vi "Reset Generator.vi"(8 "error in (no error)":errorcluster, 10 "Waveform Generation (0:1)":u16(ring) items=["1", "2"], 11 "VISA resource name":refnum<visa-resource-name>) -> (0 "error out":errorcluster, 3 "VISA resource name out":refnum<visa-resource-name>)   [LabVIEW 2015, in "Agilent 2000 3000 X-Series.lvlib"]
doc: "Restores the waveform generator factory default settings (1 kHz sine wave, 500 mVpp, 0 V offset)."
uses:
  Agilent 2000 3000 X-Series.lvlib
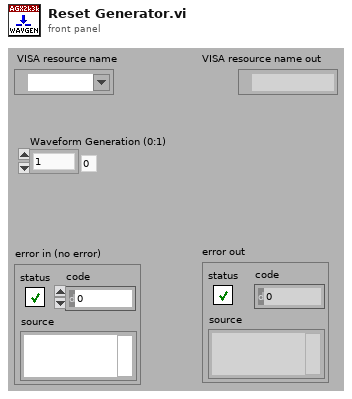
[diagram p1: front panel]
types:
  T1 = typedef "Agilent 2000 3000 X-Series.lvlib/Extended User Data.ctl" = cluster{"X-Series Mode":u16, "Acquisition Type (0: Normal)":i32}
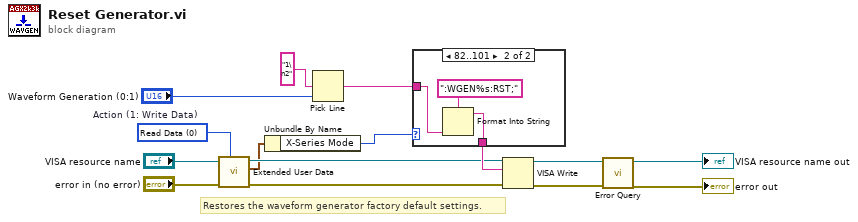
[diagram p0: block diagram]
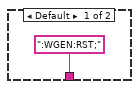
[diagram p2: hidden frame]
diagram:
  w6 = 0 items=["Read Data", "Write Data", "Clear Data", "Clear ALL Data"]  # Action (1: Write Data)
  # "Restores the waveform generator factory default settings."
  n1 = call "Extended User Data.vi"("Action (1: Write Data)"=w6, "error in (no error)"="error in (no error)", "VISA resource name in"="VISA resource name") -> ("error out"=w7:errorcluster, "User Data Out"=w5:T1, "VISA resource name out"=w8:refnum<visa-resource-name>)  [unwired: 6 in]
  n2 = Unbundle By Name(w5) -> ("X-Series Mode"=w4:u16)
  n3 = Pick Line(multi-line string="1\n2", line index="Waveform Generation (0:1)") -> (output string=w1:string)  [unwired: 1 in]
  n4 = case shown="82..101" w4 {
    tunnel: [":WGEN:RST;" w19] -> w15
    tunnel: w1 -> [_ w17]
    frame Default {
    }
    frame 82..101 {
      n5 = Format Into String(format string=":WGEN%s:RST;", w17) -> (resulting string=w19:string)  [unwired: 2 in, 1 out]
    }
  }
  n6 = VISA Write(VISA resource name=w8, write buffer=w15, error in (no error)=w7) -> (VISA resource name out=w14:refnum<visa-resource-name>, error out=w13:errorcluster)  [unwired: 1 out]
  n7 = call "Error Query.vi"("error in (no error)"=w13, "VISA resource name"=w14) -> ("error out"=→"error out":errorcluster, "VISA resource name out"=→"VISA resource name out":refnum<visa-resource-name>)  [unwired: 8 out]
